vi "disconnect.vi"(8 "error in (no error)":errorcluster, 11 "DomeController in":refnum<class "DomeController.lvclass">) -> (0 "error out":errorcluster, 3 "DomeController out":refnum<class "DomeController.lvclass">)   [LabVIEW 2016, in "DomeController.lvclass"]
uses:
  DomeController.lvclass
  DomeController.lvclass/DomeController.ctl
  domeCommunicator/ATDomeCommunicator.lvclass
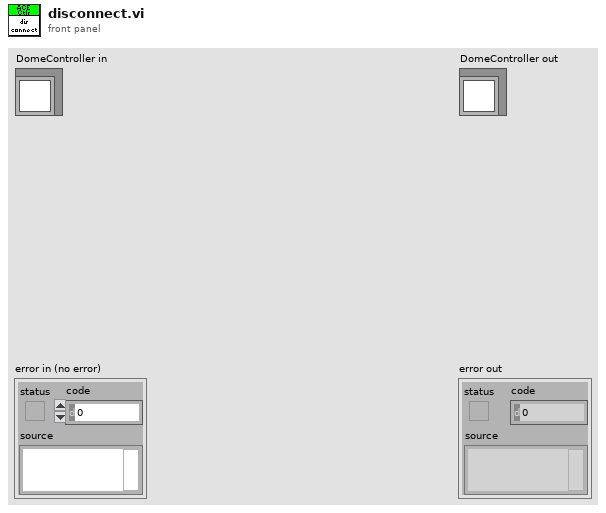
[diagram p1: front panel]
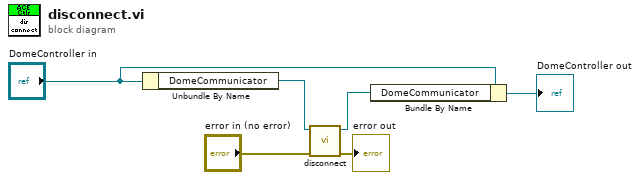
[diagram p0: block diagram]
diagram:
  n1 = Unbundle By Name("DomeController in") -> ("DomeCommunicator"=w3:refnum<class "ATDomeCommunicator.lvclass">)
  n2 = call-dynamic "disconnect.vi"("error in (no error)"="error in (no error)", "tcpDevice in"=w3) -> ("error out"=→"error out":errorcluster, "tcpDevice out"=w4:refnum<class "ATDomeCommunicator.lvclass">)  [unwired: 8 in]
  n3 = Bundle By Name(cluster="DomeController in", "DomeCommunicator"=w4) -> (→"DomeController out":refnum<class "DomeController.lvclass">)
